vi "查询上序合格.vi"(8 "error in (no error)":errorcluster, 11 "产品ID":string="123456") -> (0 "error out":errorcluster, 1 "本序已做":bool, 2 "上序合格":bool)   [LabVIEW 2013]
uses:
  <vilib>/Utility/error.llb/whitespace.ctl
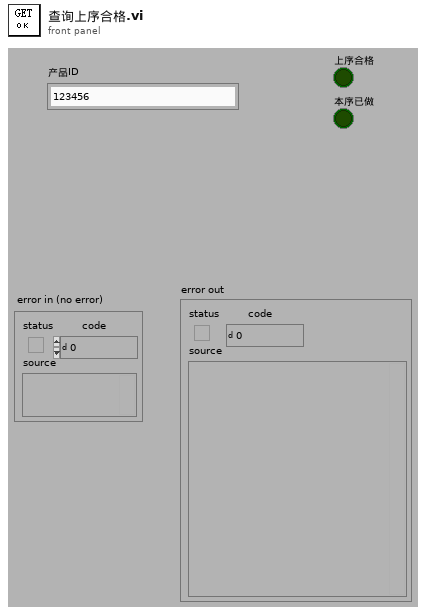
[diagram p1: front panel]
types:
  T1 = typedef "whitespace.ctl" = u16
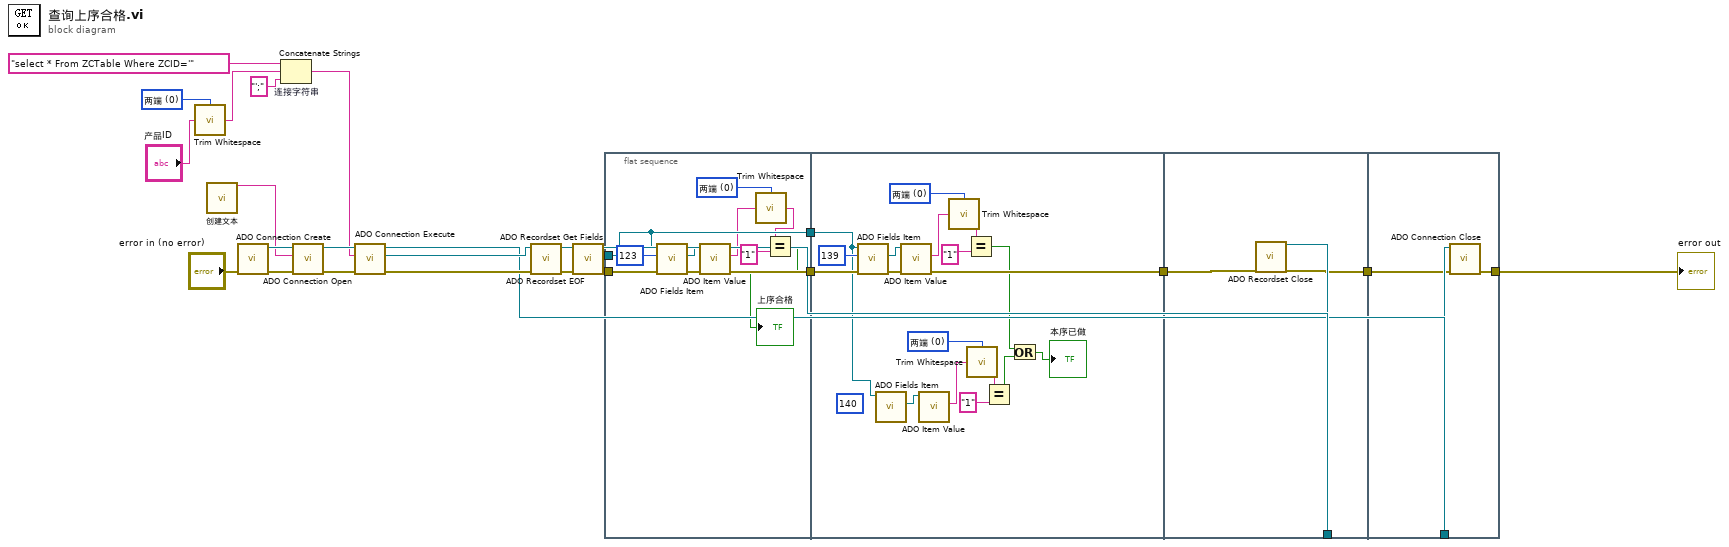
[diagram p0: block diagram]
diagram:
  w15 = T1 0 items=["两端", "字符串首端", "字符串末端"] ("location (both)")
  n1 = call <vilib>:"Trim Whitespace.vi"("string"="产品ID", "location (both)"=w15) -> ("trimmed string"=w16:string)
  n2 = call "创建文本"() -> ("Result"=w2:string)  [unwired: 14 in, 1 out]
  n3 = call "ADO Connection Create.vi"("error in (no error)"="error in (no error)") -> ("error out"=w24:errorcluster, "ADODB._Connection Out"=w25:refnum<k7>)  [unwired: 9 out]
  n4 = Concatenate Strings "连接字符串"("select * From ZCTable Where ZCID='" ("字符串 2"), w16, "';" ("字符串 2")) -> (w14:string)
  n5 = call "ADO Connection Open.vi"("error in (no error)"=w24, "ConnectionString"=w2, "ADODB._Connection In"=w25) -> ("error out"=w23:errorcluster, "ADODB._Connection Out"=w22:refnum<k7>)  [unwired: 7 out]
  n6 = call "ADO Connection Execute.vi"("error in (no error)"=w23, "CommandText"=w14, "ADODB._Connection In"=w22) -> ("error out"=w20:errorcluster, "RecordSet"=w21:refnum<k7>, "ADODB._Connection Out"=w7:refnum<k7>)  [unwired: 6 out]
  n7 = call "ADO Recordset EOF.vi"("error in (no error)"=w20, "ADODB._Recordset In"=w21) -> ("error out"=w11:errorcluster, "ADODB._Recordset Out"=w12:refnum<k7>)  [unwired: 8 out]
  n8 = call "ADO Recordset Get Fields.vi"("error in (no error)"=w11, "ADODB._Recordset In"=w12) -> ("error out"=w9:errorcluster, "Fields Out"=w10:refnum<k7>, "ADODB._Recordset Out"=w8:refnum<k7>)  [unwired: 7 out]
  n9 = flat-sequence {
    tunnel: w10 -> [w31]
    tunnel: w9 -> [w32]
    tunnel: [w36] -> w4
    tunnel: [w31] -> w3
    tunnel: w3 -> [w43]
    tunnel: w4 -> [w51]
    tunnel: [w46] -> w1
    tunnel: w8 -> [w57]
    tunnel: [w56] -> w6
    tunnel: w1 -> [w55]
    tunnel: w7 -> [w60]
    tunnel: w6 -> [w59]
    tunnel: [w58] -> w5
    frame #0 {
      w29 = T1 0 items=["两端", "字符串首端", "字符串末端"] ("location (both)")
      n10 = call "ADO Fields Item.vi"("error in (no error)"=w32, "Index"=123, "Fields In"=w31) -> ("error out"=w34:errorcluster, "Item Out"=w33:refnum<k7>)  [unwired: 7 out]
      n11 = call "ADO Item Value.vi"("error in (no error)"=w34, "Item In"=w33) -> ("error out"=w36:errorcluster, "Value"=w28:string)  [unwired: 8 out]
      n12 = call <vilib>:"Trim Whitespace.vi"("string"=w28, "location (both)"=w29) -> ("trimmed string"=w27:string)
      n13 = Equal?(x=w27, y="1") -> (x = y?=→"上序合格":bool)
    }
    frame #1 {
      w40 = T1 0 items=["两端", "字符串首端", "字符串末端"] ("location (both)")
      (unwired) 140 ("Index")
      w49 = T1 0 items=["两端", "字符串首端", "字符串末端"] ("location (both)")
      n14 = call "ADO Fields Item.vi"("error in (no error)"=w51, "Index"=139, "Fields In"=w43) -> ("error out"=w53:errorcluster, "Item Out"=w52:refnum<k7>)  [unwired: 7 out]
      n15 = call "ADO Fields Item.vi"("Fields In"=w43) -> ("Item Out"=w42:refnum<k7>)  [unwired: 2 in, 8 out]
      n16 = call "ADO Item Value.vi"("error in (no error)"=w53, "Item In"=w52) -> ("error out"=w46:errorcluster, "Value"=w48:string)  [unwired: 8 out]
      n17 = call "ADO Item Value.vi"("Item In"=w42) -> ("Value"=w41:string)  [unwired: 1 in, 9 out]
      n18 = call <vilib>:"Trim Whitespace.vi"("string"=w48, "location (both)"=w49) -> ("trimmed string"=w47:string)
      n19 = Equal?(x=w47, y="1") -> (x = y?=w37:bool)
      n20 = call <vilib>:"Trim Whitespace.vi"("string"=w41, "location (both)"=w40) -> ("trimmed string"=w44:string)
      n21 = Equal?(x=w44, y="1") -> (x = y?=w38:bool)
      n22 = Or(x=w37, y=w38) -> (x .or. y?=→"本序已做":bool)
    }
    frame #2 {
      n23 = call "ADO Recordset Close.vi"("ADODB._Recordset In"=w57, "error in (no error)"=w55) -> ("error out"=w56:errorcluster)  [unwired: 17 out]
    }
    frame #3 {
      n24 = call "ADO Connection Close.vi"("error in (no error)"=w59, "ADODB._Connection In"=w60) -> ("error out"=w58:errorcluster)  [unwired: 9 out]
    }
  }
  "error out" <- w5
